vi "Blend Colors.vi"(1 "Alpha":u8=255, 2 "Target":u32(colorbox)=16448250, 3 "Source":u32(colorbox)) -> (0 "Array":u32[](array[colorbox]))   [LabVIEW 2023, in "Font Glyph Drawer Interface.lvlib"]
uses:
  Font Glyph Drawer Interface.lvlib
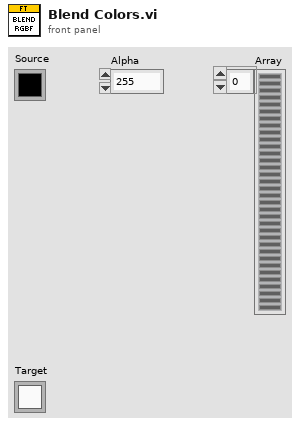
[diagram p1: front panel]
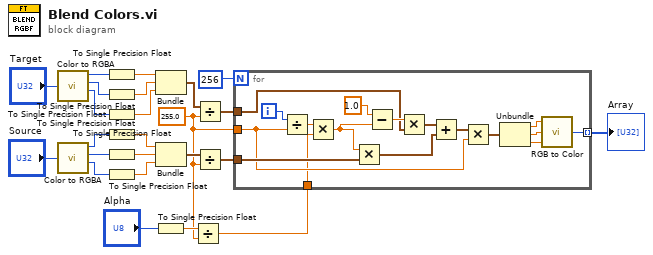
[diagram p0: block diagram]
diagram:
  w3 = sgl 255.0
  n1 = call "Color to RGBA.vi"("Color Box"="Target") -> ("R"=w11:u8, "G"=w10:u8, "B"=w9:u8)  [unwired: 1 out]
  n2 = call "Color to RGBA.vi"("Color Box"="Source") -> ("R"=w7:u8, "G"=w6:u8, "B"=w5:u8)  [unwired: 1 out]
  n3 = To Single Precision Float(number=w11) -> (single precision float=w18:sgl)
  n4 = To Single Precision Float(number=w10) -> (single precision float=w19:sgl)
  n5 = To Single Precision Float(number=w9) -> (single precision float=w20:sgl)
  n6 = To Single Precision Float(number=w7) -> (single precision float=w21:sgl)
  n7 = To Single Precision Float(number=w6) -> (single precision float=w23:sgl)
  n8 = To Single Precision Float(number=w5) -> (single precision float=w22:sgl)
  n9 = Bundle(w18, w19, w20) -> (w13:cluster{sgl, sgl, sgl})  [unwired: 1 in]
  n10 = Bundle(w21, w23, w22) -> (w14:cluster{sgl, sgl, sgl})  [unwired: 1 in]
  n11 = To Single Precision Float(number="Alpha") -> (single precision float=w4:sgl)
  n12 = Divide(x=w4, y=w3) -> (x/y=w1:sgl)
  n13 = Divide(x=w13, y=w3) -> (x/y=w15:cluster{sgl, sgl, sgl})
  n14 = Divide(x=w14, y=w3) -> (x/y=w16:cluster{sgl, sgl, sgl})
  n15 = for {
    N: 256 -> [_]
    tunnel: [w29] -> w24 mode=indexing
    tunnel: w16 -> [w38]
    tunnel: w15 -> [w36]
    tunnel: w3 -> [w27]
    tunnel: w1 -> [w25]
    i -> [w41]
    n16 = Divide(x=w41, y=w27) -> (x/y=w40:sgl)
    n17 = Multiply(x=w40, y=w25) -> (x*y=w26:sgl)
    n18 = Multiply(x=w26, y=w38) -> (x*y=w34:cluster{sgl, sgl, sgl})
    n19 = Subtract(x=sgl 1.0, y=w26) -> (x-y=w37:sgl)
    n20 = Multiply(x=w37, y=w36) -> (x*y=w35:cluster{sgl, sgl, sgl})
    n21 = Add(x=w35, y=w34) -> (x+y=w33:cluster{sgl, sgl, sgl})
    n22 = Multiply(x=w33, y=w27) -> (x*y=w28:cluster{sgl, sgl, sgl})
    n23 = Unbundle(w28) -> (w32:sgl, w31:sgl, w30:sgl)
    n24 = call <vilib>:"RGB to Color.vi"("B"=w30, "G"=w31, "R"=w32) -> ("Color"=w29:u32)
  }
  "Array" <- w24
